vi "Assert 32 bit or less wired to 32 bit or less Type.vi"   [LabVIEW 2017]
uses:
  f32efce0-4703-48d2-b113-244bd164b266.vi
  3dc5e7bf-c0fa-47c6-8c5f-4ae9761b3104.vi
  e6ebc59b-58cd-4b7a-a5f2-a0e4a5ee25cb.vi
  5a1d2e67-c8a7-4721-a3bf-e7df91e2f542.vi
  3e0b5dcd-d856-4869-941a-03074b7bc41e.vi
  eca23347-5497-43b4-94af-ed5bf14f2a90.vi
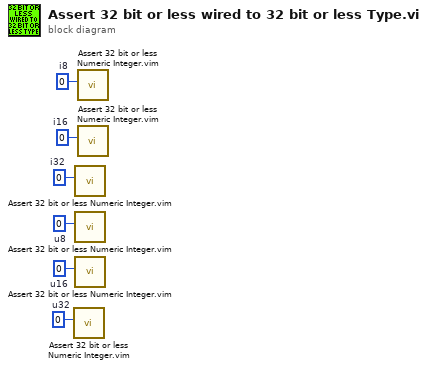
[diagram p0: block diagram]
diagram:
  w1 = u32 0  # u32
  w2 = u16 0  # u16
  w3 = u8 0  # u8
  w4 = 0  # i32
  w5 = i16 0  # i16
  w6 = i8 0  # i8
  n1 = call "Assert 32 bit or less Numeric Integer.vim"("Item in"=w1) -> ()  [unwired: 10 in, 1 out]
  n2 = call "Assert 32 bit or less Numeric Integer.vim"("Item in"=w4) -> ()  [unwired: 10 in, 1 out]
  n3 = call "Assert 32 bit or less Numeric Integer.vim"("Item in"=w3) -> ()  [unwired: 10 in, 1 out]
  n4 = call "Assert 32 bit or less Numeric Integer.vim"("Item in"=w2) -> ()  [unwired: 10 in, 1 out]
  n5 = call "Assert 32 bit or less Numeric Integer.vim"("Item in"=w6) -> ()  [unwired: 10 in, 1 out]
  n6 = call "Assert 32 bit or less Numeric Integer.vim"("Item in"=w5) -> ()  [unwired: 10 in, 1 out]
